vi "ReadConfigData.vi"(3 "ConfigData":T1) -> ()   [LabVIEW 2015, in "AppConfig.lvlib"]
uses:
  AppConfig.lvlib
  ConfigData.ctl
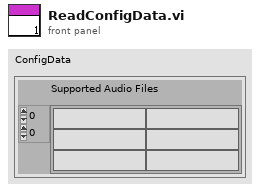
[diagram p1: front panel]
types:
  T1 = typedef "AppConfig.lvlib/ConfigData.ctl" = cluster{"Supported Audio Files":string[][]}
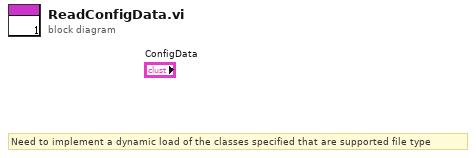
[diagram p0: block diagram]
diagram:
  # "Need to implement a dynamic load of the classes specified that are supported file type"
